vi "T13.vi"(2 "Parametry Ziemi":T1={"a - półoś duża"=6378137.0, "b - półoś mała"=6356752.3141999999998} {"b - półoś mała" format="%_20f"; "a - półoś duża" format="%_20g"}, 3 "fi'":ext) -> (7 "T13":ext)   [LabVIEW 2012, in "Biblioteka moduł map v3.lvlib" / "Konwersja wsp.lvlib" / "UTM.lvlib" / "Konwersja z UTM na wsp geograficzne.lvlib"]
uses:
  Konwersja z UTM na wsp geograficzne.lvlib
  UTM.lvlib
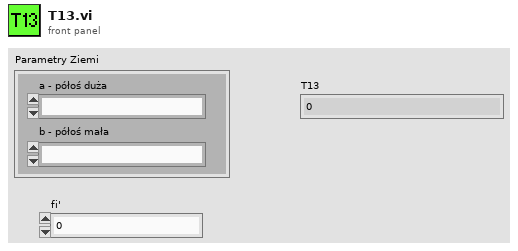
[diagram p1: front panel]
types:
  T1 = cluster{"a - półoś duża":ext, "b - półoś mała":ext}
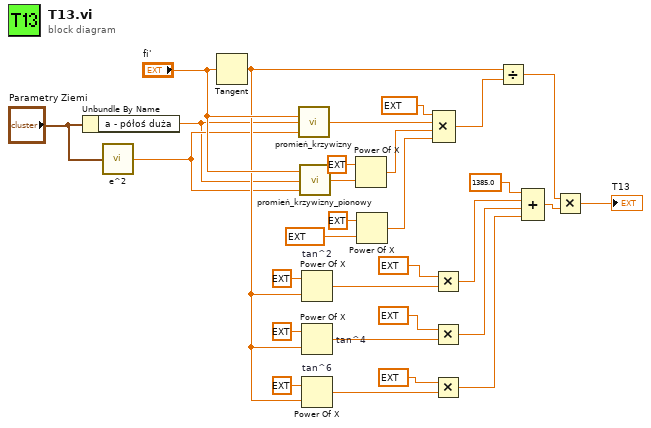
[diagram p0: block diagram]
diagram:
  n1 = Unbundle By Name("Parametry Ziemi") -> ("a - półoś duża"=w1:ext)
  n2 = call "e^2.vi"("Parametry Ziemi"="Parametry Ziemi") -> ("e^2"=w3:ext)  [unwired: 4 in]
  n3 = Tangent(1:"fi'") -> (0:w11:ext)
  n4 = call "promień_krzywizny.vi"("e^2"=w3, "a"=w1, "fi[rad]"="fi'") -> ("Promien krzywizny południka"=w28:ext)  [unwired: 2 in]
  n5 = call "promień_krzywizny_pionowy.vi"("e^2"=w3, "a"=w1, "fi[rad]"="fi'") -> ("Promien krzywizny równoleżnika"=w27:ext)  [unwired: 2 in]
  n6 = Power Of X "tan^2"(1:w11, 2:ext 2.0 ("y")) -> (0:w12:ext)
  n7 = Power Of X "tan^4"(1:w11, 2:ext 4.0 ("y")) -> (0:w8:ext)
  n8 = Power Of X "tan^6"(1:w11, 2:ext 6.0 ("y")) -> (0:w7:ext)
  n9 = Power Of X(1:w27, 2:ext 7.0 ("y")) -> (0:w23:ext)
  n10 = Power Of X(1:ext 0.9996 ("k0"), 2:ext 8.0 ("y")) -> (0:w22:ext)
  n11 = Compound Arithmetic op=MULTIPLY(ext 40320.0 ("value"), w28, w23, w22) -> (w30:ext)
  n12 = Multiply(x=ext 3633.0, y=w12) -> (x*y=w13:ext)
  n13 = Multiply(x=ext 4095.0, y=w8) -> (x*y=w6:ext)
  n14 = Multiply(x=ext 1575.0, y=w7) -> (x*y=w5:ext)
  n15 = Divide(x=w11, y=w30) -> (x/y=w21:ext)
  n16 = Compound Arithmetic op=ADD(1385.0 ("value"), w13, w6, w5) -> (w19:ext)
  n17 = Multiply(x=w21, y=w19) -> (x*y=→"T13":ext)
